vi "Design a Floating-Point Filter Part 1.vi"   [LabVIEW 2023]
doc: "Part 1 of the Designing a Floating-Point Filter tutorial."
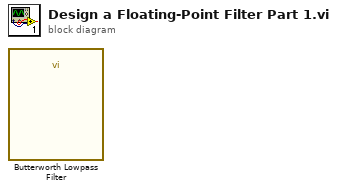
[diagram p0: block diagram]
diagram:
  n1 = call "Butterworth Lowpass Filter"() -> ()  [unwired: 1 in, 11 out]
